vi "disablebuttons.vi"(8 "error in (no error)":errorcluster, 10 "Disabled":T1(ring), 11 "Front Panel References":refnum<vi>[](array[refnum])) -> (0 "error out":errorcluster)   [LabVIEW 2017]
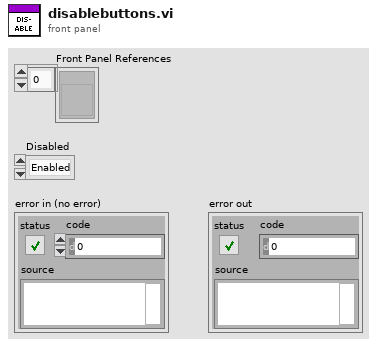
[diagram p1: front panel]
types:
  T1 = enum8{"Enabled", "Disabled", "Disabled and Grayed Out"}
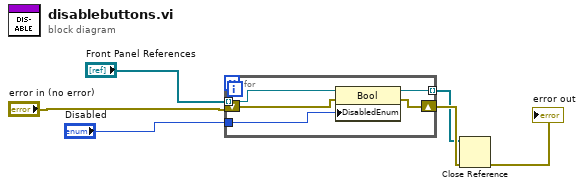
[diagram p0: block diagram]
diagram:
  n1 = for {
    tunnel: "Front Panel References" -> [w11] mode=indexing
    tunnel: "Disabled" -> [w10]
    shift-right: [w8] -> w5
    shift-left: "error in (no error)" -> [w9]
    tunnel: [w7] -> w4 mode=indexing
    n2 = property on="Property Node" class="Bool"(reference=w11, error in=w9, "DisabledEnum"=w10) -> (reference out=w7:refnum<vi>, error out=w8:errorcluster)
  }
  n3 = Close Reference(reference=w4, error in (no error)=w5) -> (error out=→"error out":errorcluster)
